vi "ModuFPGA_dark.vi"() -> ()   [LabVIEW 2012]
uses:
  <vilib>/Platform/TimedLoop/XDataNode/timing_clust.ctl
  <vilib>/Platform/TimedLoop/XDataNode/nitl_modes.ctl
  <vilib>/Platform/TimedLoop/XDataNode/wakeup.ctl
  <vilib>/rvi/DataTransferAndStorage/Container/Common/niFpgaContainerMetaDataKey.ctl
  <vilib>/rvi/DataTransferAndStorage/Container/Common/niFpgaContainerState.ctl
  <vilib>/rvi/DataTransferAndStorage/Container/Common/niFpgaDataTypeControl.ctl
  <vilib>/rvi/DataTransferAndStorage/Container/Common/niFpgaContainerImplementationControl.ctl
  <vilib>/rvi/DataTransferAndStorage/Container/Common/niFpgaContainerArbitrationOptionsControl.ctl
  <vilib>/rvi/DataTransferAndStorage/Container/Common/niFpgaTransferTypeControl.ctl
  <vilib>/rvi/DataTransferAndStorage/Container/Common/niFpgaContainerInitializationParameters.ctl
  <vilib>/rvi/Memory/Memory_Types/niFpgaMemoryInterfaceConfiguration.ctl
  <vilib>/rvi/FIFO/Fifo_Types/niFpgaFifoControlLogicControl.ctl
  <vilib>/rvi/eio/common/nirviEmuTemplateMethod_errors.vi
  <vilib>/rvi/FIFO/Fifo_Resource/nirvififoEmulationSetSize.vi
  <vilib>/rvi/DataTransferAndStorage/Container/Common/niFpgaContainerGetUniqueNameForEmu.vi
  <vilib>/rvi/Emulation/niFpgaSctlEmulationRegisterWithScheduler.vi
  <vilib>/rvi/Emulation/niFpgaSctlEmulationScheduler.vi
  <vilib>/rvi/DataTransferAndStorage/Container/Common/niFpgaContainerSetEmuInfo.vi
  <vilib>/rvi/eio/common/nirviEmuReportErrorAndStop.vi
  <vilib>/rvi/Emulation/niFpgaSctlEmulationFifoFullMgr.vi
  <vilib>/rvi/errors/niFpgaSetErrorForExecOnDevCompSimple.vi
  <vilib>/rvi/Memory/Memory_Emulation/niFpgaMemoryEmulationCacheClearOnFirstRun.vi
  <vilib>/rvi/Memory/Memory_Emulation/nirvimemoryEmulationManagerCache_MakeExclusive.vi
  <vilib>/rvi/Memory/Memory_Emulation/niFpgaMemoryEmulationValidateCache.vi
  <vilib>/rvi/Memory/Memory_Emulation/nirvimemoryEmulationManagerCache_ReleaseExclusive.vi
  <vilib>/rvi/Memory/Memory_Emulation/nirvimemoryEmulationManagerCache_InsertValue.vi
  <vilib>/Utility/error.llb/Clear Errors.vi
  <vilib>/rvi/Memory/Memory_Emulation/nirvimemoryEmulationManagerCache_GetValue.vi
  <vilib>/rvi/Emulation/niFpgaSctlEmulationResourceMgr.vi
  <vilib>/eio/EIONode/EIONode.xnode
  <vilib>/Platform/TimedLoop/XDataNode/XDataNode.xnode
  <vilib>/rvi/DataTransferAndStorage/Container/XNode/niFpgaContainer.xnode
  <vilib>/rvi/FIFO/Fifo_Resource/nirvififoEmulationClear.vi
  <vilib>/rvi/LocalResourceManager/LocalResourceManager.xnode
  <vilib>/rvi/FIFO/Fifo_Resource/nirvififoEmulationRead.vi
  <vilib>/rvi/Memory/Memory_Emulation/nirvimemoryEmulation.vi
  <vilib>/rvi/FIFO/Fifo_Resource/nirvififoEmulationWrite.vi
  <vilib>/Platform/TimedLoop/XDataNode/XDNodeRunTimeDep.lvlib
panel:
  out "IO Module\\ADC Error A":bool
  out "IO Module\\ADC Error B":bool
  out "IO Module\\Pll Unlocked":bool
  in  "Record Size only data":u32=95
  out "DMA FIFO Timed Out?":bool
  in  "circular buffer length":u32=1000
  in  "location":i16(ring) items=["Purdue", "NIKHEF", "Zurich", "???"]
  in  "Trigger 0":i16=4000
  in  "Trigger 1":i16=4000
  in  "Trigger 2":i16=4000
  in  "Trigger 3":i16=4000
  in  "Trigger 4":i16=4000
  in  "Trigger 5":i16=4000
  in  "Trigger 6":i16=4000
  in  "Trigger 7":i16=4000
  in  "# of pretrigger":u32=20
  in  "initial value":u64
  in  "channel 0 on/off":bool
  in  "channel 2 on/off":bool
  in  "channel 1 on/off":bool
  in  "channel 3 on/off":bool
  in  "channel 4 on/off":bool
  in  "channel 5 on/off":bool
  in  "channel 6 on/off":bool
  in  "channel 7 on/off":bool
  in  "Testpulse duration (20 ns ticks)":u32=1
  in  "Testpulse Separation (20 ns ticks)":u32=500
  in  "Testpulse Time Delay (20 ns ticks)":u32=15
  in  "Testpulser On/Off":bool
  out "Init Done":bool
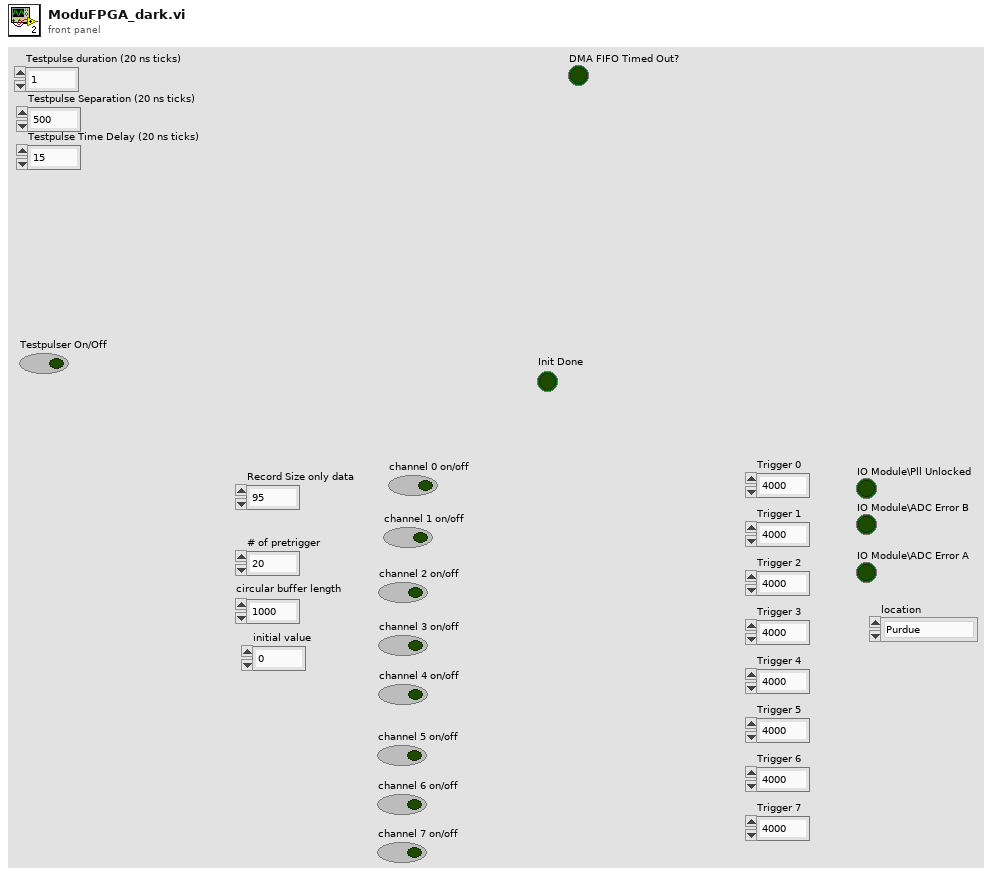
[diagram p1: front panel]
types:
  T1 = typedef "XDNodeRunTimeDep.lvlib/timing_clust.ctl" = cluster{"Expected End [f-1]":u64, "Actual End [f-1]":u64, "Finished Late? [f-1]":bool, "Expected End [i-1]":u64, "Actual End [i-1]":u64, "Finished Late? [i-1]":bool, "Expected Start [i]":u64, "Actual Start [i]":u64, "Expected Start [f]":u64, "Actual Start [f]":u64, "Source Name":string, "Structure Name":string, "Period":i64, "Deadline":i64, "Offset":i64, "Start":i64, "Priority":i32, "Timeout":i32, "Mode":T2, "Wakeup Reason":T3, "Error":errorcluster, "Source Type":string, "Secondary Source Type":string, "Global End Time":u64, "Global Start Time":u64, "Frame Duration":u64, "Iteration Duration":u64, "Assigned CPU":i32, "I/O Scan Engine Mode":u32}
  T2 = typedef "XDNodeRunTimeDep.lvlib/nitl_modes.ctl" = enum32{"No Change", "Process missed periods, maintain original phase", "Discard missed periods, maintain original phase", "Process missed periods, ignore original phase", "Discard missed periods, ignore original phase"}
  T3 = typedef "XDNodeRunTimeDep.lvlib/wakeup.ctl" = enum32{"Normal", "Aborted", "Asynchronous wakeup", "Timing source error", "Timed loop error", "Timeout"}
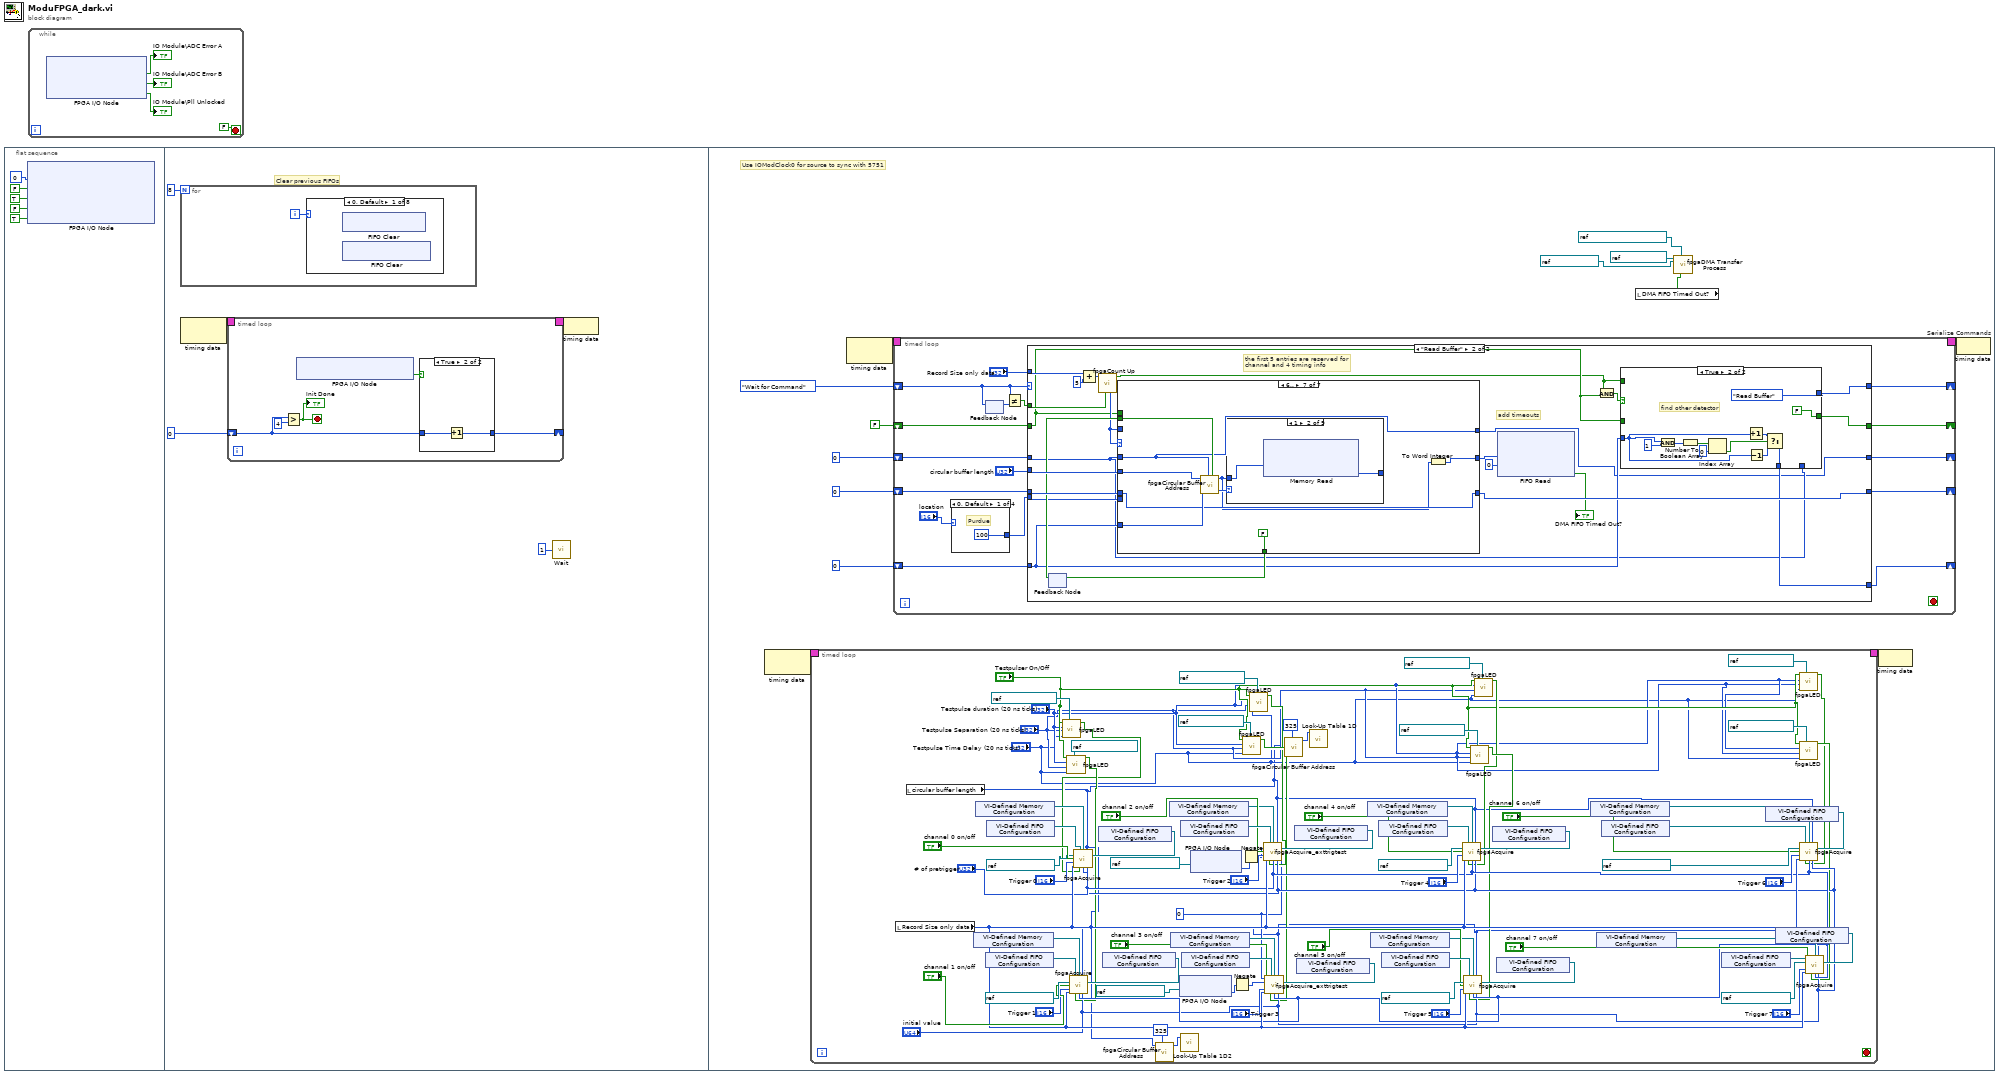
[diagram p0: block diagram]
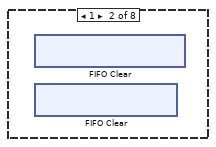
[diagram p2: hidden frame]
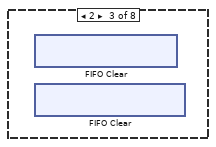
[diagram p3: hidden frame]
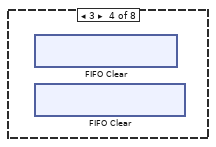
[diagram p4: hidden frame]
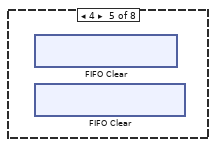
[diagram p5: hidden frame]
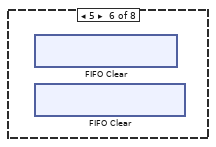
[diagram p6: hidden frame]
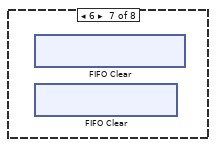
[diagram p7: hidden frame]
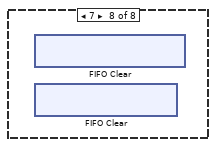
[diagram p8: hidden frame]
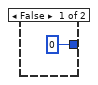
[diagram p9: hidden frame]
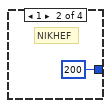
[diagram p10: hidden frame]
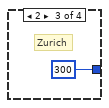
[diagram p11: hidden frame]
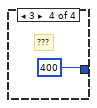
[diagram p12: hidden frame]
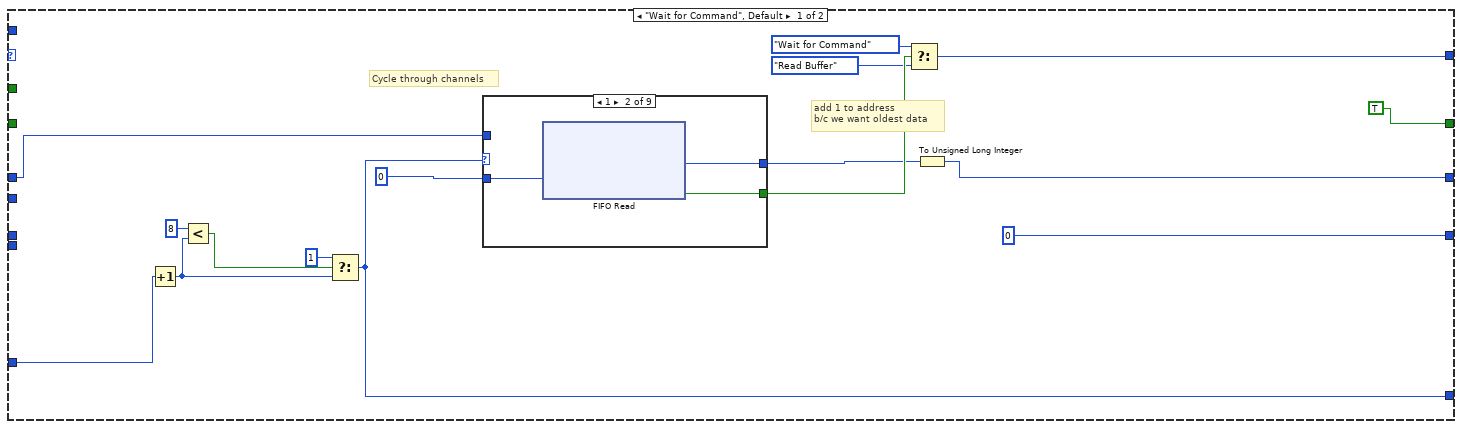
[diagram p13: hidden frame]
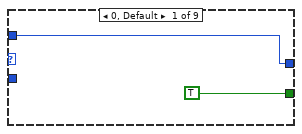
[diagram p14: hidden frame]
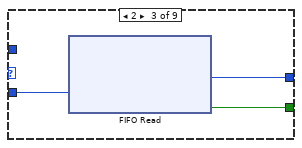
[diagram p15: hidden frame]
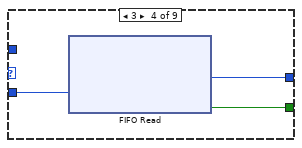
[diagram p16: hidden frame]
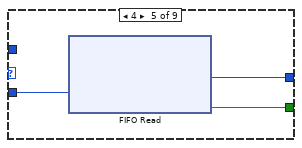
[diagram p17: hidden frame]
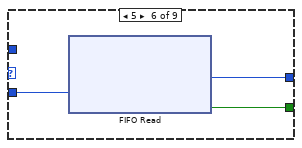
[diagram p18: hidden frame]
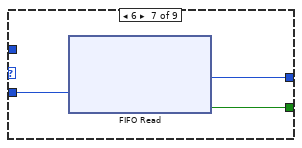
[diagram p19: hidden frame]
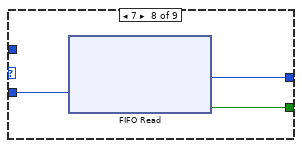
[diagram p20: hidden frame]
diagram:
  n1 = flat-sequence {
    frame #0 {
      n2 = xnode "FPGA I/O Node"("IO Module\\Sample Clock Select"=u8 0 ("IO Module\\Sample Clock Select"), "IO Module\\Force Initialization"=FALSE ("IO Module\\Force Initialization"), "IO Module\\Force Initialization"=TRUE ("IO Module\\Force Initialization"), "IO Module\\Force Initialization"=FALSE ("IO Module\\Force Initialization"), "IO Module\\Digital Output Enable"=TRUE ("IO Module\\Digital Output Enable")) -> ()  [unwired: 5 in, 5 out]
    }
    frame #1 {
      # "Clear previous FIFOs"
      n3 = for {
        N: 8 -> [_]
        i -> [w11]
        n4 = case shown="0, Default" w11 {
          frame 0, Default {
            n5 = xnode ("FIFO Clear")() -> ()  [unwired: 1 in, 1 out]
            n6 = xnode ("FIFO Clear")() -> ()  [unwired: 1 in, 1 out]
          }
          frame 1 {
            n7 = xnode ("FIFO Clear")() -> ()  [unwired: 1 in, 1 out]
            n8 = xnode ("FIFO Clear")() -> ()  [unwired: 1 in, 1 out]
          }
          frame 2 {
            n9 = xnode ("FIFO Clear")() -> ()  [unwired: 1 in, 1 out]
            n10 = xnode ("FIFO Clear")() -> ()  [unwired: 1 in, 1 out]
          }
          frame 3 {
            n11 = xnode ("FIFO Clear")() -> ()  [unwired: 1 in, 1 out]
            n12 = xnode ("FIFO Clear")() -> ()  [unwired: 1 in, 1 out]
          }
          frame 4 {
            n13 = xnode ("FIFO Clear")() -> ()  [unwired: 1 in, 1 out]
            n14 = xnode ("FIFO Clear")() -> ()  [unwired: 1 in, 1 out]
          }
          frame 5 {
            n15 = xnode ("FIFO Clear")() -> ()  [unwired: 1 in, 1 out]
            n16 = xnode ("FIFO Clear")() -> ()  [unwired: 1 in, 1 out]
          }
          frame 6 {
            n17 = xnode ("FIFO Clear")() -> ()  [unwired: 1 in, 1 out]
            n18 = xnode ("FIFO Clear")() -> ()  [unwired: 1 in, 1 out]
          }
          frame 7 {
            n19 = xnode ("FIFO Clear")() -> ()  [unwired: 1 in, 1 out]
            n20 = xnode ("FIFO Clear")() -> ()  [unwired: 1 in, 1 out]
          }
        }
      }
      n21 = node-c288() -> (w10:T1)  [unwired: 1 in]
      n22 = timed-loop {
        shift-right: [w15] -> _
        shift-left: u16 0 -> [w14]
        timing: w10 -> [_]
        timing-out: [_] -> w9
        stop <- w12 stop-if-true
        n23 = Greater?(x=w14, y=u16 4) -> (0:w12:bool)
        "Init Done" <- w12
        n24 = xnode "FPGA I/O Node"() -> ("IO Module\\Initialization Done"=w16:bool)  [unwired: 1 in, 1 out]
        n25 = case shown="True" w16 {
          tunnel: [u16 0 w19] -> w15
          tunnel: w14 -> [_ w18]
          frame False {
          }
          frame True {
            n26 = Increment(x=w18) -> (x+1=w19:u16)
          }
        }
      }
      n27 = call "Wait"("Count(mSec)"=u32 1) -> ()  [unwired: 1 out]
      n28 = node-c288(w9) -> ()
    }
    frame #2 {
      # "Use IOModClock0 for source to sync with 5751"
      n29 = node-c288() -> (w30:T1)  [unwired: 1 in]
      n30 = timed-loop {
        timing: w30 -> [_]
        timing-out: [_] -> w29
        stop <- _ stop-if-true
        w44 = i16 0
        n31 = local read "Record Size only data"() -> (w95:u32)
        n32 = local read "circular buffer length"() -> (w37:u32)
        n33 = xnode "VI-Defined Memory Configuration"() -> ("Memory Out"=w71:refnum<k21>)
        n34 = xnode "VI-Defined Memory Configuration"() -> ("Memory Out"=w78:refnum<k21>)
        n35 = xnode "VI-Defined FIFO Configuration"() -> ("FIFO Out"=w117:refnum<k21>)
        n36 = xnode "VI-Defined FIFO Configuration"() -> ("FIFO Out"=w96:refnum<k21>)
        n37 = call "fpgaLED.vi"("FPGA I/O In"=refnum<k21> "IO Module\\D0 0", "Testpulse Time Delay (20 ns ticks)"="Testpulse Time Delay (20 ns ticks)", "Testpulse Separation (20 ns ticks)"="Testpulse Separation (20 ns ticks)", "Testpulse duration (20 ns ticks)"="Testpulse duration (20 ns ticks)", "Testpulser On/Off"="Testpulser On/Off") -> ("Is Test Pulse?"=w53:bool)  [unwired: 5 in, 1 out]
        n38 = call "fpgaLED.vi"("FPGA I/O In"=refnum<k21> "IO Module\\D0 1", "Testpulse Time Delay (20 ns ticks)"="Testpulse Time Delay (20 ns ticks)", "Testpulse Separation (20 ns ticks)"="Testpulse Separation (20 ns ticks)", "Testpulse duration (20 ns ticks)"="Testpulse duration (20 ns ticks)", "Testpulser On/Off"="Testpulser On/Off") -> ("Is Test Pulse?"=w54:bool)  [unwired: 5 in, 1 out]
        n39 = xnode "VI-Defined FIFO Configuration"() -> ("FIFO Out"=w69:refnum<k21>)
        n40 = call "fpgaAcquire.vi"("Command FIFO"=w96, "Circular Buffer Mem"=w78, "circular buffer length"=w37, "FPGA I/O In"=refnum<k21> "IO Module\\AI A0", "Timing FIFO"=w69, "channel on/off"="channel 0 on/off", "Trigger"="Trigger 0", "Samples to Acquire"=w95, "Is Test Pulse?"=w53, "# of pretrigger"="# of pretrigger", "timing"="initial value") -> ()  [unwired: 5 in]
        n41 = xnode "VI-Defined FIFO Configuration"() -> ("FIFO Out"=w70:refnum<k21>)
        n42 = call "fpgaAcquire.vi"("Command FIFO"=w117, "Circular Buffer Mem"=w71, "circular buffer length"=w37, "FPGA I/O In"=refnum<k21> "IO Module\\AI A1", "Timing FIFO"=w70, "channel on/off"="channel 1 on/off", "Trigger"="Trigger 1", "Samples to Acquire"=w95, "Is Test Pulse?"=w54, "# of pretrigger"="# of pretrigger", "timing"="initial value") -> ()  [unwired: 5 in]
        n43 = call "fpgaCircular Buffer Address.vi"("Starting Address"=u32 325, "circular buffer length"=w37) -> ("Address"=w45:u32)  [unwired: 9 in]
        n44 = xnode "VI-Defined Memory Configuration"() -> ("Memory Out"=w77:refnum<k21>)
        n45 = xnode "VI-Defined Memory Configuration"() -> ("Memory Out"=w72:refnum<k21>)
        n46 = xnode "FPGA I/O Node"("FPGA I/O In"=refnum<k21> "IO Module\\AI A3") -> ("I/O Item"=w43:i16)  [unwired: 1 out]
        n47 = xnode "VI-Defined FIFO Configuration"() -> ("FIFO Out"=w115:refnum<k21>)
        n48 = call "Look-Up Table 1D2"("address"=w45) -> ()  [unwired: 8 in, 1 out]
        n49 = xnode "VI-Defined FIFO Configuration"() -> ("FIFO Out"=w116:refnum<k21>)
        n50 = xnode "FPGA I/O Node"("FPGA I/O In"=refnum<k21> "IO Module\\AI A2") -> ("I/O Item"=w39:i16)  [unwired: 1 out]
        n51 = Negate(x=w43) -> (-x=w42:i16)
        n52 = Negate(x=w39) -> (-x=w38:i16)
        n53 = call "fpgaLED.vi"("FPGA I/O In"=refnum<k21> "IO Module\\D0 3", "Testpulse Time Delay (20 ns ticks)"="Testpulse Time Delay (20 ns ticks)", "Testpulse Separation (20 ns ticks)"="Testpulse Separation (20 ns ticks)", "Testpulse duration (20 ns ticks)"="Testpulse duration (20 ns ticks)", "Testpulser On/Off"="Testpulser On/Off") -> ("Is Test Pulse?"=w56:bool)  [unwired: 5 in, 1 out]
        n54 = call "fpgaLED.vi"("FPGA I/O In"=refnum<k21> "IO Module\\D0 2", "Testpulse Time Delay (20 ns ticks)"="Testpulse Time Delay (20 ns ticks)", "Testpulse Separation (20 ns ticks)"="Testpulse Separation (20 ns ticks)", "Testpulse duration (20 ns ticks)"="Testpulse duration (20 ns ticks)", "Testpulser On/Off"="Testpulser On/Off") -> ("Is Test Pulse?"=w55:bool)  [unwired: 5 in, 1 out]
        n55 = call "fpgaCircular Buffer Address.vi"("Starting Address"=u32 325, "circular buffer length"=w37) -> ("Address"=w47:u32)  [unwired: 9 in]
        n56 = xnode "VI-Defined FIFO Configuration"() -> ("FIFO Out"=w68:refnum<k21>)
        n57 = call "fpgaAcquire_exttrigtest.vi"("Starting Address"=w44, "Command FIFO"=w115, "Circular Buffer Mem"=w77, "circular buffer length"=w37, "Fake data in"=w38, "Timing FIFO"=w68, "channel on/off"="channel 2 on/off", "Trigger"="Trigger 2", "Samples to Acquire"=w95, "Is Test Pulse?"=w55, "# of pretrigger"="# of pretrigger", "timing"="initial value") -> ()  [unwired: 4 in]
        n58 = xnode "VI-Defined FIFO Configuration"() -> ("FIFO Out"=w67:refnum<k21>)
        n59 = call "fpgaAcquire_exttrigtest.vi"("Starting Address"=w44, "Command FIFO"=w116, "Circular Buffer Mem"=w72, "circular buffer length"=w37, "Fake data in"=w42, "Timing FIFO"=w67, "channel on/off"="channel 3 on/off", "Trigger"="Trigger 3", "Samples to Acquire"=w95, "Is Test Pulse?"=w56, "# of pretrigger"="# of pretrigger", "timing"="initial value") -> ()  [unwired: 4 in]
        n60 = call "Look-Up Table 1D"("address"=w47) -> ()  [unwired: 8 in, 1 out]
        n61 = xnode "VI-Defined Memory Configuration"() -> ("Memory Out"=w76:refnum<k21>)
        n62 = xnode "VI-Defined Memory Configuration"() -> ("Memory Out"=w73:refnum<k21>)
        n63 = xnode "VI-Defined FIFO Configuration"() -> ("FIFO Out"=w111:refnum<k21>)
        n64 = xnode "VI-Defined FIFO Configuration"() -> ("FIFO Out"=w112:refnum<k21>)
        n65 = call "fpgaLED.vi"("FPGA I/O In"=refnum<k21> "IO Module\\D0 5", "Testpulse Time Delay (20 ns ticks)"="Testpulse Time Delay (20 ns ticks)", "Testpulse Separation (20 ns ticks)"="Testpulse Separation (20 ns ticks)", "Testpulse duration (20 ns ticks)"="Testpulse duration (20 ns ticks)", "Testpulser On/Off"="Testpulser On/Off") -> ("Is Test Pulse?"=w58:bool)  [unwired: 5 in, 1 out]
        n66 = call "fpgaLED.vi"("FPGA I/O In"=refnum<k21> "IO Module\\D0 4", "Testpulse Time Delay (20 ns ticks)"="Testpulse Time Delay (20 ns ticks)", "Testpulse Separation (20 ns ticks)"="Testpulse Separation (20 ns ticks)", "Testpulse duration (20 ns ticks)"="Testpulse duration (20 ns ticks)", "Testpulser On/Off"="Testpulser On/Off") -> ("Is Test Pulse?"=w57:bool)  [unwired: 5 in, 1 out]
        n67 = xnode "VI-Defined FIFO Configuration"() -> ("FIFO Out"=w63:refnum<k21>)
        n68 = call "fpgaAcquire.vi"("Command FIFO"=w111, "Circular Buffer Mem"=w76, "circular buffer length"=w37, "FPGA I/O In"=refnum<k21> "IO Module\\AI A4", "Timing FIFO"=w63, "channel on/off"="channel 4 on/off", "Trigger"="Trigger 4", "Samples to Acquire"=w95, "Is Test Pulse?"=w57, "# of pretrigger"="# of pretrigger", "timing"="initial value") -> ()  [unwired: 5 in]
        n69 = xnode "VI-Defined FIFO Configuration"() -> ("FIFO Out"=w66:refnum<k21>)
        n70 = call "fpgaAcquire.vi"("Command FIFO"=w112, "Circular Buffer Mem"=w73, "circular buffer length"=w37, "FPGA I/O In"=refnum<k21> "IO Module\\AI A5", "Timing FIFO"=w66, "channel on/off"="channel 5 on/off", "Trigger"="Trigger 5", "Samples to Acquire"=w95, "Is Test Pulse?"=w58, "# of pretrigger"="# of pretrigger", "timing"="initial value") -> ()  [unwired: 5 in]
        n71 = xnode "VI-Defined Memory Configuration"() -> ("Memory Out"=w75:refnum<k21>)
        n72 = xnode "VI-Defined Memory Configuration"() -> ("Memory Out"=w74:refnum<k21>)
        n73 = xnode "VI-Defined FIFO Configuration"() -> ("FIFO Out"=w114:refnum<k21>)
        n74 = xnode "VI-Defined FIFO Configuration"() -> ("FIFO Out"=w113:refnum<k21>)
        n75 = xnode "VI-Defined FIFO Configuration"() -> ("FIFO Out"=w64:refnum<k21>)
        n76 = xnode "VI-Defined FIFO Configuration"() -> ("FIFO Out"=w65:refnum<k21>)
        n77 = call "fpgaLED.vi"("FPGA I/O In"=refnum<k21> "IO Module\\D0 6", "Testpulse Time Delay (20 ns ticks)"="Testpulse Time Delay (20 ns ticks)", "Testpulse Separation (20 ns ticks)"="Testpulse Separation (20 ns ticks)", "Testpulse duration (20 ns ticks)"="Testpulse duration (20 ns ticks)", "Testpulser On/Off"="Testpulser On/Off") -> ("Is Test Pulse?"=w59:bool)  [unwired: 5 in, 1 out]
        n78 = call "fpgaLED.vi"("FPGA I/O In"=refnum<k21> "IO Module\\D0 7", "Testpulse Time Delay (20 ns ticks)"="Testpulse Time Delay (20 ns ticks)", "Testpulse Separation (20 ns ticks)"="Testpulse Separation (20 ns ticks)", "Testpulse duration (20 ns ticks)"="Testpulse duration (20 ns ticks)", "Testpulser On/Off"="Testpulser On/Off") -> ("Is Test Pulse?"=w60:bool)  [unwired: 5 in, 1 out]
        n79 = call "fpgaAcquire.vi"("Command FIFO"=w114, "Circular Buffer Mem"=w75, "circular buffer length"=w37, "FPGA I/O In"=refnum<k21> "IO Module\\AI A6", "Timing FIFO"=w64, "channel on/off"="channel 6 on/off", "Trigger"="Trigger 6", "Samples to Acquire"=w95, "Is Test Pulse?"=w59, "# of pretrigger"="# of pretrigger", "timing"="initial value") -> ()  [unwired: 5 in]
        n80 = call "fpgaAcquire.vi"("Command FIFO"=w113, "Circular Buffer Mem"=w74, "circular buffer length"=w37, "FPGA I/O In"=refnum<k21> "IO Module\\AI A7", "Timing FIFO"=w65, "channel on/off"="channel 7 on/off", "Trigger"="Trigger 7", "Samples to Acquire"=w95, "Is Test Pulse?"=w60, "# of pretrigger"="# of pretrigger", "timing"="initial value") -> ()  [unwired: 5 in]
      }
      n81 = node-c288() -> (w32:T1)  [unwired: 1 in]
      n82 = timed-loop "Serialize Commands" {
        timing: w32 -> [_]
        timing-out: [_] -> w31
        shift-right: [w708] -> _
        shift-left: enum16{"Wait for Command", "Read Buffer"}."Wait for Command" -> [w706]
        shift-right: [w712] -> _
        shift-left: u32 0 ("Element") -> [w711]
        shift-right: [w710] -> _
        shift-left: u8 0 ("t") -> [w709]
        shift-right: [w703] -> _
        shift-left: u64 0 ("Element") -> [w702]
        shift-right: [w698] -> _
        shift-left: FALSE -> [w699]
        stop <- _ stop-if-true
        n83 = case shown="0, Default" "location" {
          tunnel: [i16 100 i16 200 i16 300 i16 400] -> w700
          frame 0, Default {
            # "Purdue"
          }
          frame 1 {
            # "NIKHEF"
          }
          frame 2 {
            # "Zurich"
          }
          frame 3 {
            # "???"
          }
        }
        n84 = feedback-in #1(w706) -> ()
        n85 = feedback #1() -> (w707:enum16{"Wait for Command", "Read Buffer"})  [unwired: 1 in]
        n86 = Not Equal?(x=w706, y=w707) -> (x != y?=w704:bool)
        n87 = case shown="\"Read Buffer\"" w706 {
          tunnel: "Record Size only data" -> [_ w778]
          tunnel: [w722 w764] -> w710
          tunnel: w709 -> [w724 w769]
          tunnel: [w725 w760] -> w712
          tunnel: w711 -> [w718 w761]
          tunnel: [w728 w766] -> w708
          tunnel: "circular buffer length" -> [_ w782]
          tunnel: w704 -> [_ w779]
          tunnel: [u64 0 ("Element") w775] -> w703
          tunnel: w702 -> [_ w774]
          tunnel: w700 -> [_ w770]
          tunnel: w699 -> [_ w763]
          tunnel: [TRUE w767] -> w698
          frame "Wait for Command", Default {
            # "add 1 to address\nb/c we want oldest data"
            # "Cycle through channels"
            n88 = Increment(x=w724) -> (x+1=w723:u8)
            n89 = Less?(x=u8 8, y=w723) -> (x < y?=w732:bool)
            n90 = Select(t=u8 1, s=w732, f=w723) -> (s? t:f=w722:u8)
            n91 = case shown="1" w722 {
              tunnel: [TRUE ("Timed Out?") w738 w739 w742 w745 w748 w751 w754 w757] -> w729
              tunnel: 0 ("Timeout") -> [_ w736 w741 w744 w747 w750 w753 w756 w759]
              tunnel: [w734 w737 w740 w743 w746 w749 w752 w755 w758] -> w721
              tunnel: w718 -> [w734 _ _ _ _ _ _ _ _]
              frame 0, Default {
              }
              frame 1 {
                n92 = xnode ("FIFO Read")("Timeout"=w736) -> ("Element"=w737:i16, "Timed Out?"=w738:bool)  [unwired: 1 in, 1 out]
              }
              frame 2 {
                n93 = xnode ("FIFO Read")("Timeout"=w741) -> ("Element"=w740:i16, "Timed Out?"=w739:bool)  [unwired: 1 in, 1 out]
              }
              frame 3 {
                n94 = xnode ("FIFO Read")("Timeout"=w744) -> ("Element"=w743:i16, "Timed Out?"=w742:bool)  [unwired: 1 in, 1 out]
              }
              frame 4 {
                n95 = xnode ("FIFO Read")("Timeout"=w747) -> ("Element"=w746:i16, "Timed Out?"=w745:bool)  [unwired: 1 in, 1 out]
              }
              frame 5 {
                n96 = xnode ("FIFO Read")("Timeout"=w750) -> ("Element"=w749:i16, "Timed Out?"=w748:bool)  [unwired: 1 in, 1 out]
              }
              frame 6 {
                n97 = xnode ("FIFO Read")("Timeout"=w753) -> ("Element"=w752:i16, "Timed Out?"=w751:bool)  [unwired: 1 in, 1 out]
              }
              frame 7 {
                n98 = xnode ("FIFO Read")("Timeout"=w756) -> ("Element"=w755:i16, "Timed Out?"=w754:bool)  [unwired: 1 in, 1 out]
              }
              frame 8 {
                n99 = xnode ("FIFO Read")("Timeout"=w759) -> ("Element"=w758:i16, "Timed Out?"=w757:bool)  [unwired: 1 in, 1 out]
              }
            }
            n100 = Select(t=enum16{"Wait for Command", "Read Buffer"}."Wait for Command", s=w729, f=enum16{"Wait for Command", "Read Buffer"}."Read Buffer") -> (s? t:f=w728:enum16{"Wait for Command", "Read Buffer"})
            n101 = To Unsigned Long Integer(number=w721) -> (unsigned 32bit integer=w725:u32)
          }
          frame "Read Buffer" {
            # "the first 5 entries are reserved for channel and 4 timing info"
            # "add timeouts"
            n102 = feedback #2() -> (w773:bool)  [unwired: 1 in]
            n103 = Add(x=w778, y=u32 5) -> (x+y=w776:u32)
            n104 = call "fpgaCount Up.vi"("Reset?"=w779, "goal"=w776) -> ("Count Met"=w762:bool, "count"=w765:u32)  [unwired: 8 in]
            n105 = case shown="6.." w765 {
              tunnel: w769 -> [_ w810 w824 _ _ _ w870]
              tunnel: w761 -> [_ w813 w826 w850 w856 w862 w868]
              tunnel: w782 -> [_ _ _ _ _ _ w873]
              tunnel: [i16 0 ("Data") w811 w828 w848 w854 w860 w867] -> w780
              tunnel: w773 -> [_ _ _ _ _ _ w872]
              tunnel: [u64 0 ("Element") w804 w825 w851 w857 w863 w869] -> w775
              tunnel: w774 -> [_ w804 w820 w851 w857 w863 w869]
              tunnel: [u32 0 ("Element") w813 w826 w850 w856 w862 w868] -> w760
              tunnel: [FALSE FALSE FALSE FALSE FALSE TRUE FALSE] -> w772
              tunnel: w770 -> [_ w806 _ _ _ _ _]
              tunnel: w763 -> [_ w805 w821 _ _ _ _]
              tunnel: w765 -> [_ _ _ _ _ _ _]
              frame 0, Default {
              }
              frame 1 {
                n106 = Decrement(x=w810) -> (x-1=w809:u8)
                n107 = To Word Integer(number=w809) -> (16bit integer=w808:i16)
                n108 = Add(x=w806, y=w808) -> (x+y=w807:i16)
                n109 = case shown="False" w805 {
                  tunnel: [w814 w818] -> w811
                  tunnel: w807 -> [w815 w817]
                  frame False {
                    w816 = u16 2 items=["Header Information", "Particle Pulse", "Test Pulse"] ("Pulse Type")
                    # "is not the trigger"
                    n110 = call "fpgaBit Manipulation.vi"("Pulse Type"=w816, "Integer to be written"=w815) -> ("Integer Written"=w814:i16)  [unwired: 2 in]
                  }
                  frame True {
                    w819 = u16 0 items=["Header Information", "Particle Pulse", "Test Pulse"] ("Pulse Type")
                    # "is the trigger"
                    n111 = call "fpgaBit Manipulation.vi"("Pulse Type"=w819, "Integer to be written"=w817) -> ("Integer Written"=w818:i16)  [unwired: 2 in]
                  }
                }
              }
              frame 2 {
                # "reads out the lsb of the timing information"
                n112 = case shown="True" w821 {
                  tunnel: [w829 w831] -> w825
                  tunnel: w824 -> [_ w830]
                  tunnel: w820 -> [w829 _]
                  frame False {
                  }
                  frame True {
                    n113 = case shown="1" w830 {
                      tunnel: [_ w832 w834 w836 w838 w840 w842 w844 w846] -> w831
                      frame Default {
                      }
                      frame 1 {
                        n114 = xnode ("FIFO Read")("Timeout"=0) -> ("Element"=w832:u64)  [unwired: 1 in, 2 out]
                      }
                      frame 2 {
                        n115 = xnode ("FIFO Read")("Timeout"=0) -> ("Element"=w834:u64)  [unwired: 1 in, 2 out]
                      }
                      frame 3 {
                        n116 = xnode ("FIFO Read")("Timeout"=0) -> ("Element"=w836:u64)  [unwired: 1 in, 2 out]
                      }
                      frame 4 {
                        n117 = xnode ("FIFO Read")("Timeout"=0) -> ("Element"=w838:u64)  [unwired: 1 in, 2 out]
                      }
                      frame 5 {
                        n118 = xnode ("FIFO Read")("Timeout"=0) -> ("Element"=w840:u64)  [unwired: 1 in, 2 out]
                      }
                      frame 6 {
                        n119 = xnode ("FIFO Read")("Timeout"=0) -> ("Element"=w842:u64)  [unwired: 1 in, 2 out]
                      }
                      frame 7 {
                        n120 = xnode ("FIFO Read")("Timeout"=0) -> ("Element"=w844:u64)  [unwired: 1 in, 2 out]
                      }
                      frame 8 {
                        n121 = xnode ("FIFO Read")("Timeout"=0) -> ("Element"=w846:u64)  [unwired: 1 in, 2 out]
                      }
                    }
                  }
                }
                n122 = Split Number(x=w825) -> (hi(x)=w823:u32)  [unwired: 1 out]
                n123 = Split Number(x=w823) -> (hi(x)=w822:u16)  [unwired: 1 out]
                n124 = To Word Integer(number=w822) -> (16bit integer=w828:i16)
              }
              frame 3 {
                n125 = Split Number(x=w851) -> (hi(x)=w853:u32)  [unwired: 1 out]
                n126 = Split Number(x=w853) -> (lo(x)=w852:u16)  [unwired: 1 out]
                n127 = To Word Integer(number=w852) -> (16bit integer=w848:i16)
              }
              frame 4 {
                n128 = Split Number(x=w857) -> (lo(x)=w859:u32)  [unwired: 1 out]
                n129 = Split Number(x=w859) -> (hi(x)=w858:u16)  [unwired: 1 out]
                n130 = To Word Integer(number=w858) -> (16bit integer=w854:i16)
              }
              frame 5 {
                n131 = Split Number(x=w863) -> (lo(x)=w865:u32)  [unwired: 1 out]
                n132 = Split Number(x=w865) -> (lo(x)=w864:u16)  [unwired: 1 out]
                n133 = To Word Integer(number=w864) -> (16bit integer=w860:i16)
              }
              frame 6.. {
                n134 = call "fpgaCircular Buffer Address.vi"("Reset?"=w872, "Starting Address"=w868, "circular buffer length"=w873) -> ("Address"=w866:u32)  [unwired: 8 in]
                n135 = case shown="1" w870 {
                  tunnel: w866 -> [_ w876 w878 w880 w882 w884 w886 w888 w890]
                  tunnel: [i16 0 w875 w877 w879 w881 w883 w885 w887 w889] -> _
                  frame Default {
                    # "Error"
                  }
                  frame 1 {
                    n136 = xnode ("Memory Read")("Address"=w876) -> ("Data"=w875:i16)  [unwired: 1 in, 1 out]
                  }
                  frame 2 {
                    n137 = xnode ("Memory Read")("Address"=w878) -> ("Data"=w877:i16)  [unwired: 1 in, 1 out]
                  }
                  frame 3 {
                    n138 = xnode ("Memory Read")("Address"=w880) -> ("Data"=w879:i16)  [unwired: 1 in, 1 out]
                  }
                  frame 4 {
                    n139 = xnode ("Memory Read")("Address"=w882) -> ("Data"=w881:i16)  [unwired: 1 in, 1 out]
                  }
                  frame 5 {
                    n140 = xnode ("Memory Read")("Address"=w884) -> ("Data"=w883:i16)  [unwired: 1 in, 1 out]
                  }
                  frame 6 {
                    n141 = xnode ("Memory Read")("Address"=w886) -> ("Data"=w885:i16)  [unwired: 1 in, 1 out]
                  }
                  frame 7 {
                    n142 = xnode ("Memory Read")("Address"=w888) -> ("Data"=w887:i16)  [unwired: 1 in, 1 out]
                  }
                  frame 8 {
                    n143 = xnode ("Memory Read")("Address"=w890) -> ("Data"=w889:i16)  [unwired: 1 in, 1 out]
                  }
                }
                n144 = To Word Integer(number=w866) -> (16bit integer=w867:i16)
              }
            }
            n145 = feedback-in #2(w772) -> ()
            n146 = xnode ("FIFO Read")("Element"=w780, "Timeout"=0) -> ("Timed Out?"=→"DMA FIFO Timed Out?":bool)  [unwired: 1 in, 1 out]
            n147 = And(x=w762, y=w763) -> (x .and. y?=w768:bool)
            n148 = case shown="True" w768 {
              tunnel: w769 -> [w784 w790]
              tunnel: [w788 FALSE] -> w767
              tunnel: w763 -> [w788 _]
              tunnel: [w785 enum16{"Wait for Command", "Read Buffer"}."Read Buffer"] -> w766
              tunnel: [w784 w789] -> w764
              tunnel: w762 -> [w783 _]
              tunnel: w761 -> [_ _]
              frame False {
                n149 = Select(t=enum16{"Wait for Command", "Read Buffer"}."Wait for Command", s=w783, f=enum16{"Wait for Command", "Read Buffer"}."Read Buffer") -> (s? t:f=w785:enum16{"Wait for Command", "Read Buffer"})
              }
              frame True {
                # "find other detector"
                n150 = And(x=w790, y=u8 1) -> (x .and. y?=w795:u8)
                n151 = Number To Boolean Array(number=w795) -> (Boolean array=w794:bool[])
                n152 = Index Array(array=w794, index=0) -> (element=w792:bool)
                n153 = Increment(x=w790) -> (x+1=w798:u8)
                n154 = Decrement(x=w790) -> (x-1=w797:u8)
                n155 = Select(t=w798, s=w792, f=w797) -> (s? t:f=w789:u8)
              }
            }
          }
        }
      }
      n156 = local read "DMA FIFO Timed Out?"() -> (w33:bool)
      n157 = call "fpgaDMA Transfer Process.vi"("DMA Write Timed Out?"=w33, "Clock Domain"=refnum<k21> "40 MHz Onboard Clock", "Local"=refnum<k21> "To DMA FIFO", "DMA"=refnum<k21> "To Host FIFO") -> ()  [unwired: 8 in]
      n158 = node-c288(w29) -> ()
      n159 = node-c288(w31) -> ()
    }
  }
  n160 = while {
    stop <- FALSE stop-if-true
    n161 = xnode "FPGA I/O Node"() -> ("IO Module\\ADC Error A"=→"IO Module\\ADC Error A":bool, "IO Module\\ADC Error B"=→"IO Module\\ADC Error B":bool, "IO Module\\Pll Unlocked"=→"IO Module\\Pll Unlocked":bool)  [unwired: 3 in, 3 out]
  }
